vi "InitImg.vi"(8 "error in (no error)":errorcluster, 11 "EpiWrapper in":refnum<class "EpiWrapper.lvclass">) -> (0 "error out":errorcluster, 3 "EpiWrapper out":refnum<class "EpiWrapper.lvclass">)   [LabVIEW 2012, in "EpiWrapper.lvclass"]
uses:
  EpiWrapper.lvclass
  Controls/Waferimage.ctl
  EpiWrapper.lvclass/EpiWrapper.ctl
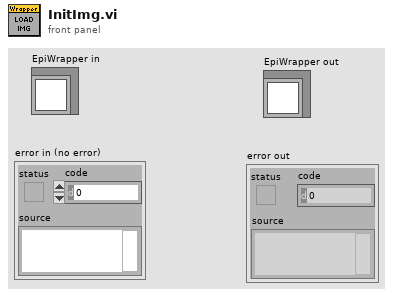
[diagram p1: front panel]
types:
  T1 = typedef "Waferimage.ctl" = picture
  T2 = typedef "LVBoundsTypeDef.ctl" = cluster{"Width":u32, "Height":u32}
  T3 = typedef "imagedata.ctl" = cluster{"image type":i32, "image depth":i32, "image":u8[], "mask":u8[], "colors":u32[], "Rectangle":cluster{"left":i16, "top":i16, "right":i16, "bottom":i16}}
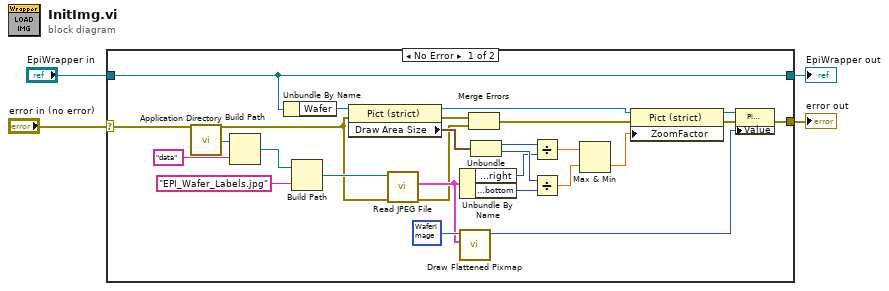
[diagram p0: block diagram]
diagram:
  n1 = case shown="No Error" "error in (no error)" {
    selector: "error in (no error)" -> [w6 w32]
    tunnel: [w8 w32] -> w3
    tunnel: [w5 w31] -> w1
    tunnel: "EpiWrapper in" -> [w5 w31]
    frame No Error {
      n2 = call <vilib>:"Application Directory.vi"() -> ("Application Directory"=w29:path)
      n3 = Build Path(base path=w29, name or relative path="data") -> (appended path=w11:path)
      n4 = Unbundle By Name(w5) -> ("Wafer"=w7:refnum<vi>)
      n5 = Build Path(base path=w11, name or relative path="EPI_Wafer_Labels.jpg") -> (appended path=w9:path)
      n6 = property class="Pict (strict)"(reference=w7, error in=w6) -> (reference out=w19:refnum<vi>, error out=w16:errorcluster, "Draw Area Size"=w20:T2)
      n7 = call <vilib>:"Read JPEG File.vi"("error in (no error)"=w6, "path to JPEG file"=w9) -> ("error out"=w17:errorcluster, "image data"=w28:T3)  [unwired: 7 in, 1 out]
      n8 = Unbundle By Name(w28) -> ("Rectangle.right"=w24:i16, "Rectangle.bottom"=w25:i16)
      n9 = call <vilib>:"Draw Flattened Pixmap.vi"("image data"=w28, "picture"=T1 bytes[544710] ("Wafer")) -> ("new picture"=w21:picture)  [unwired: 7 in]
      n10 = Merge Errors(w16, w17) -> (w15:errorcluster)
      n11 = Unbundle(w20) -> ("Width"=w27:u32, "Height"=w26:u32)
      n12 = Divide(x=w27, y=w24) -> (x/y=w23:dbl)
      n13 = Divide(x=w26, y=w25) -> (x/y=w22:dbl)
      n14 = Max & Min(x=w23, y=w22) -> (min(x,y)=w18:dbl)  [unwired: 1 out]
      n15 = property class="Pict (strict)"(reference=w19, error in=w15, "ZoomFactor"=w18) -> (reference out=w14:refnum<vi>, error out=w13:errorcluster)
      n16 = property class="Pict (strict)"(reference=w14, error in=w13, "Value"=w21) -> (error out=w8:errorcluster)  [unwired: 1 out]
    }
    frame Error {
    }
  }
  "error out" <- w3
  "EpiWrapper out" <- w1
